vi "Create Queues.vi"(8 "error in (no error)":errorcluster, 11 "Socket in":refnum<class "Socket.lvclass">) -> (0 "error out":errorcluster, 3 "Socket out":refnum<class "Socket.lvclass">)   [LabVIEW 2018, in "Socket.lvclass"]
uses:
  Socket.lvclass
  Socket.lvclass/Socket.ctl
  RxTx/CM_RxTx.lvclass
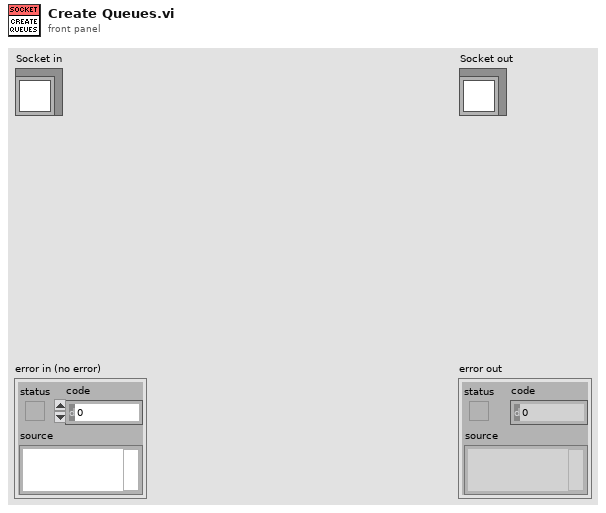
[diagram p1: front panel]
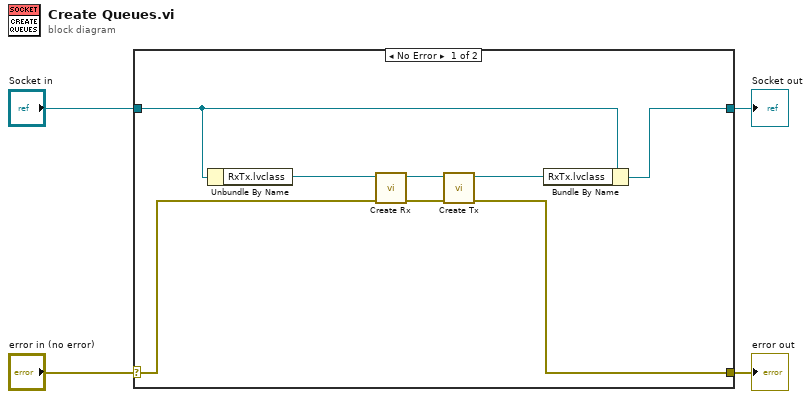
[diagram p0: block diagram]
diagram:
  n1 = case shown="No Error" "error in (no error)" {
    selector: "error in (no error)" -> [w7 w14]
    tunnel: [w5 w14] -> w3
    tunnel: [w11 w13] -> w1
    tunnel: "Socket in" -> [w12 w13]
    frame No Error {
      n2 = Unbundle By Name(w12) -> ("RxTx.lvclass"=w10:refnum<class "CM_RxTx.lvclass">)
      n3 = call "Create Rx.vi"("error in (no error)"=w7, "RxTx in"=w10) -> ("error out"=w6:errorcluster, "RxTx out"=w9:refnum<class "CM_RxTx.lvclass">)  [unwired: 8 in]
      n4 = call "Create Tx.vi"("error in (no error)"=w6, "RxTx in"=w9) -> ("error out"=w5:errorcluster, "RxTx out"=w8:refnum<class "CM_RxTx.lvclass">)  [unwired: 8 in]
      n5 = Bundle By Name(cluster=w12, "RxTx.lvclass"=w8) -> (w11:refnum<class "Socket.lvclass">)
    }
    frame Error {
    }
  }
  "error out" <- w3
  "Socket out" <- w1
